vi "nivsfpga_GetFpgaTargetClass.vi"(0 "FPGA target":refnum<vi>) -> (1 "Target":string, 2 "Platform":string)   [LabVIEW 2010]
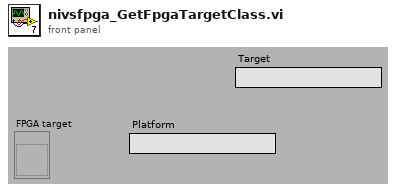
[diagram p1: front panel]
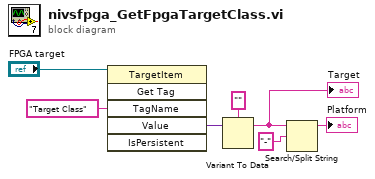
[diagram p0: block diagram]
diagram:
  n1 = invoke class="TargetItem" method="Get Tag"(reference="FPGA target", "TagName"="Target Class" ("Tag Name")) -> ("Value"=w6:variant)  [unwired: 4 in, 5 out]
  n2 = Variant To Data(Variant=w6, type="") -> (data=w2:string)  [unwired: 1 in, 1 out]
  "Target" <- w2
  n3 = Search/Split String(string=w2, search string/char (-)="-" ("string")) -> (substring before match=→"Platform":string)  [unwired: 1 in, 2 out]
